vi "IMAQdx Snap.vi"(8 "error in":errorcluster, 10 "Image In":T2, 11 "Session In":T1) -> (0 "error out":errorcluster, 2 "Image Out":T2, 3 "Session Out":T1)   [LabVIEW 2020, in "NI_Vision_Acquisition_Software.lvlib"]
doc: "Configures, starts, acquires, and unconfigures a snap acquisition. Use a snap for low-speed or single-capture applications where ease of programming is essential. If you call this VI before calling the IMAQdx Open Camera VI, the IMAQdx Snap VI uses cam0 by default. If the image type does not match the video format of the camera, this VI changes the image type to a suitable format."
uses:
  NI_Vision_Acquisition_Software.lvlib
  IMAQdx.ctl
  IMAQ Image.ctl
  IMAQdx Acquisition Mode.ctl
  IMAQdx Buffer Number Mode.ctl
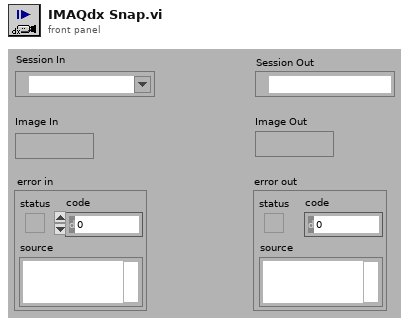
[diagram p1: front panel]
types:
  T1 = typedef "IMAQdx.ctl" = refnum<k21>
  T2 = typedef "IMAQ Image.ctl" = refnum<image>
  T3 = typedef "NI_Vision_Acquisition_Software.lvlib/IMAQdx Buffer Number Mode.ctl" = enum32{"Next", "Last", "Buffer Number", "Every", "Last New"}
  T4 = typedef "NI_Vision_Acquisition_Software.lvlib/IMAQdx Acquisition Mode.ctl" = enum32{"One Shot", "Continuous"}
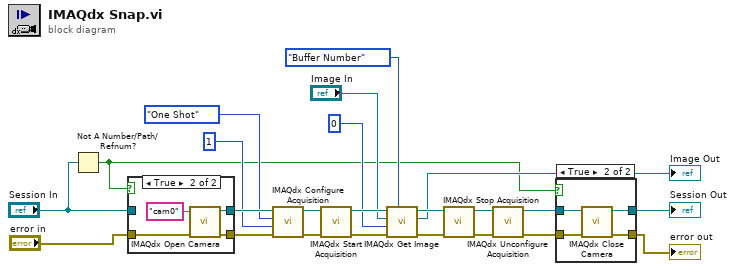
[diagram p0: block diagram]
diagram:
  n1 = Not A Number/Path/Refnum?(number/path/refnum="Session In") -> (NaN/Path/Refnum?=w3:bool)
  n2 = case shown="True" w3 {
    tunnel: [w25 w29] -> w23
    tunnel: "Session In" -> [w25 _]
    tunnel: [w24 w28] -> w21
    tunnel: "error in" -> [w24 w27]
    frame False {
    }
    frame True {
      n3 = call "IMAQdx Open Camera.vi"("error in"=w27, "Session In"="cam0") -> ("error out"=w28:errorcluster, "Session Out"=w29:T1)  [unwired: 8 in]
    }
  }
  n4 = call "IMAQdx Configure Acquisition.vi"("error in"=w21, "Number of Buffers"=u32 1, "Continuous?"=IMAQdx_Acquisition_Mode."One Shot", "Session In"=w23) -> ("error out"=w16:errorcluster, "Session Out"=w17:T1)  [unwired: 6 in]
  n5 = call "IMAQdx Start Acquisition.vi"("error in"=w16, "Session In"=w17) -> ("error out"=w14:errorcluster, "Session Out"=w15:T1)  [unwired: 8 in]
  n6 = call "IMAQdx Get Image.vi"("Buffer Number Mode (Next)"=IMAQdx_Buffer_Number_Mode."Buffer Number" ("Buffer Number Mode"), "error in"=w14, "Buffer Number In"=u32 0, "Image In"="Image In", "Session In"=w15) -> ("error out"=w9:errorcluster, "Image Out"=→"Image Out":T2, "Session Out"=w10:T1)  [unwired: 3 in, 1 out]
  n7 = call "IMAQdx Stop Acquisition.vi"("error in"=w9, "Session In"=w10) -> ("error out"=w6:errorcluster, "Session Out"=w7:T1)  [unwired: 8 in]
  n8 = call "IMAQdx Unconfigure Acquisition.vi"("error in"=w6, "Session In"=w7) -> ("error out"=w5:errorcluster, "Session Out"=w4:T1)  [unwired: 8 in]
  n9 = case shown="True" w3 {
    tunnel: w5 -> [w30 w34]
    tunnel: w4 -> [w31 w32]
    tunnel: [w31 w32] -> w2
    tunnel: [w30 w33] -> w1
    frame False {
    }
    frame True {
      n10 = call "IMAQdx Close Camera.vi"("error in"=w34, "Session In"=w32) -> ("error out"=w33:errorcluster)  [unwired: 9 in]
    }
  }
  "Session Out" <- w2
  "error out" <- w1
